vi "样品上电.vi"(6 "error in (no error)":errorcluster, 9 "仪器实例 out":T1) -> (0 "error out":errorcluster, 3 "仪器实例 out 2":T1)   [LabVIEW 2020]
uses:
  F:/F020/S7_1200 control/HslCommunication.dll
  S7_1200 control/HslCommunication.dll
  S7_1200 control/S7_1200 WriteBools.vi
  <instrlib>/TDK-Lambda G Series/TDK-Lambda G Series.lvlib
  S7_1200 control/S7_1200 control.lvlib
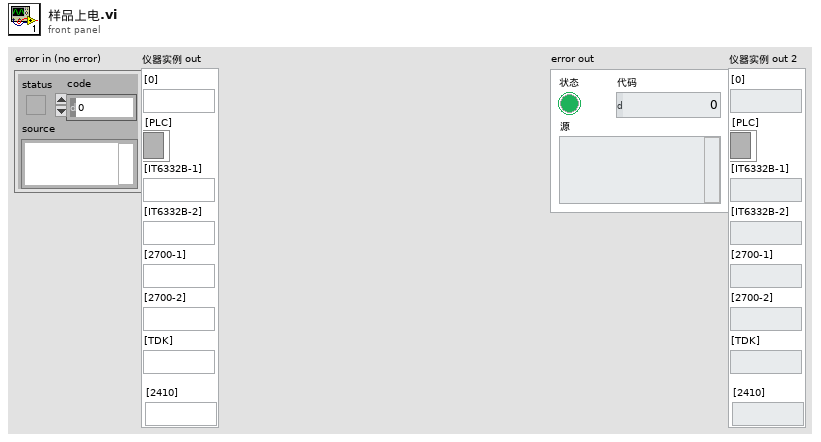
[diagram p1: front panel]
types:
  T1 = typedef "仪器实例.ctl" = cluster{"[0]":string, "[PLC]":refnum<k24>, "[IT6332B-1]":string, "[IT6332B-2]":string, "[2700-1]":string, "[2700-2]":string, "[TDK]":string, "[2410]":string}
  T2 = cluster{"Channel1":bool, "Channel2":bool, "Channel3":bool}
  T3 = cluster{"Address":i16, "Baud Rate":u32, "Language Selector":i16}
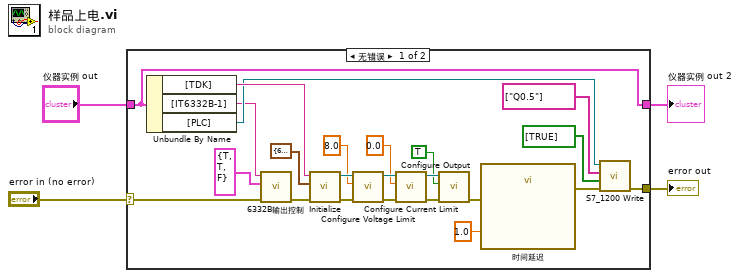
[diagram p0: block diagram]
diagram:
  n1 = case shown="无错误" "error in (no error)" {
    selector: "error in (no error)" -> [w13 w29]
    tunnel: "仪器实例 out" -> [w16 w28]
    tunnel: [w15 w29] -> w3
    tunnel: [w16 w28] -> w1
    frame No Error {
      n2 = Unbundle By Name(w16) -> ("[TDK]"=w26:string, "[IT6332B-1]"=w12:string, "[PLC]"=w14:refnum<k24>)
      n3 = call "6332B输出控制.vi"("错误输入"=w13, "Choose Channel"=T2 {"Channel1"=TRUE, "Channel2"=TRUE, "Channel3"=FALSE}, "VISA资源名称"=w12) -> ("错误输出"=w10:errorcluster)  [unwired: 7 in, 1 out]
      n4 = call <instrlib>:"Initialize.vi"("error in (no error)"=w10, "Configuration"=T3 {"Address"=6, "Baud Rate"=9600, "Language Selector"=1}, "VISA resource name"=w26) -> ("error out"=w25:errorcluster, "VISA resource name out"=w24:refnum<visa-resource-name>)  [unwired: 7 in]
      n5 = call <instrlib>:"Configure Voltage Limit.vi"("error in (no error)"=w25, "Voltage Limit (0V)"=8.0, "VISA resource name"=w24) -> ("error out"=w22:errorcluster, "VISA resource name out"=w21:refnum<visa-resource-name>)  [unwired: 7 in]
      n6 = call <instrlib>:"Configure Current Limit.vi"("error in (no error)"=w22, "Current Limit (0A)"=0.0, "VISA resource name"=w21) -> ("error out"=w18:errorcluster, "VISA resource name out"=w19:refnum<visa-resource-name>)  [unwired: 7 in]
      n7 = call <instrlib>:"Configure Output.vi"("error in (no error)"=w18, "Enable Output (False)"=TRUE, "VISA resource name"=w19) -> ("error out"=w7:errorcluster)  [unwired: 7 in, 1 out]
      n8 = call "时间延迟"("error in (no error)"=w7, "Delay Time (s)"=1.0) -> ("error out"=w6:errorcluster)  [unwired: 9 in]
      n9 = call-poly "S7_1200 Write.vi"("错误输入（无错误）"=w6, "values"=bool[] [TRUE], "addresses"=string[] ["Q0.5"], "引用"=w14) -> ("错误输出"=w15:errorcluster)  [unwired: 2 in, 1 out]
    }
    frame Error {
    }
  }
  "error out" <- w3
  "仪器实例 out 2" <- w1
